vi "RGBU32toU8.vi"(11 "RGBarrayU32":u32[][](array[numeric])) -> (3 "RGBarrayU8":u8[][][](array[numeric]))   [LabVIEW 2014]
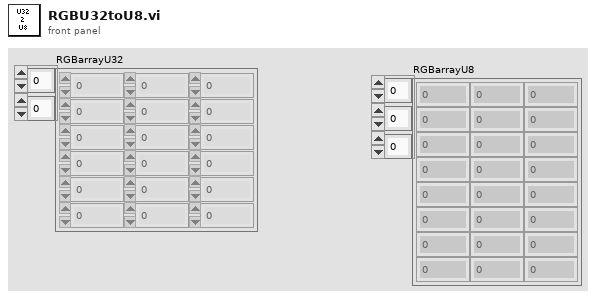
[diagram p1: front panel]
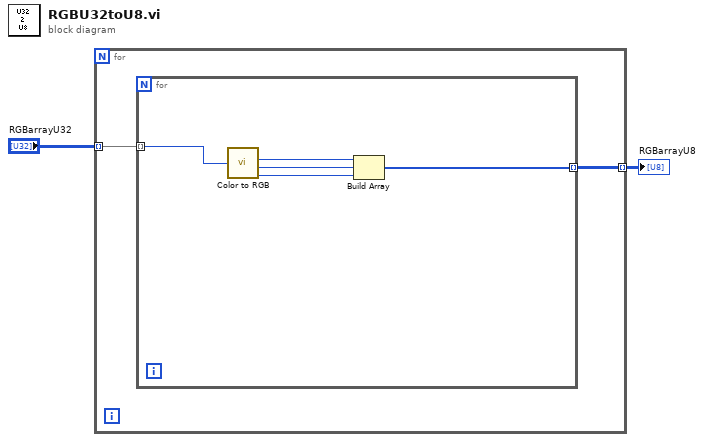
[diagram p0: block diagram]
diagram:
  n1 = for {
    tunnel: "RGBarrayU32" -> [w4] mode=indexing
    tunnel: [w3] -> w1 mode=indexing
    n2 = for {
      tunnel: w4 -> [w9] mode=indexing
      tunnel: [w5] -> w3 mode=indexing
      n3 = call <vilib>:"Color to RGB.vi"("Color"=w9) -> ("R"=w8:u8, "G"=w7:u8, "B"=w6:u8)  [unwired: 1 out]
      n4 = Build Array(w8, w7, w6) -> (w5:u8[])
    }
  }
  "RGBarrayU8" <- w1
